vi "DimIndicators.dic_info_service.vi"(0 "controlRef":refnum<vi>, 2 "serviceName":string, 5 "error in (no error)":errorcluster) -> (14 "controlRef out":refnum<vi>, 19 "error out":errorcluster)   [LabVIEW 2015, in "DimIndicators.lvlib"]
doc: "Registers a control of one of the types in \"typedefs\" to a DIM service. If no longer used, a registered event should be unregistered using \"release service\"."
uses:
  DimIndicators.lvlib
  DimIndicators.numericType.ctl
  DimIndicators.numericArrayType.ctl
  DimIndicators.anyType.ctl
  DimIndicators.dataType.ctl
  DimIndicators.actionType.ctl
panel:
  in  "anyType":T1
  in  "numericArrayType":T2
  in  "numericType":T3
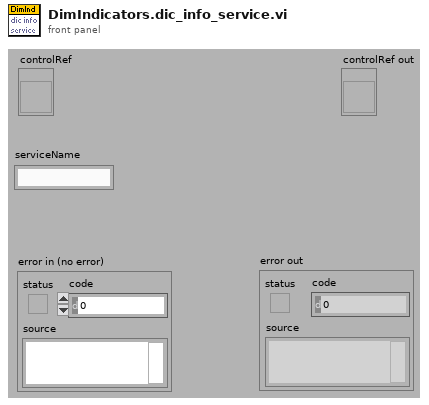
[diagram p1: front panel]
types:
  T1 = typedef "DimIndicators.lvlib/DimIndicators.anyType.ctl" = cluster{"data":string, "no link":bool, "quality":i32, "timeStamp":dbl}
  T2 = typedef "DimIndicators.lvlib/DimIndicators.numericArrayType.ctl" = cluster{"data":dbl[], "no link":bool, "quality":i32, "timeStamp":dbl}
  T3 = typedef "DimIndicators.lvlib/DimIndicators.numericType.ctl" = cluster{"data":dbl, "no link":bool, "quality":i32, "timeStamp":dbl}
  T4 = typedef "DimIndicators.lvlib/DimIndicators.dataType.ctl" = enum16{"unknown", "numeric", "numericArray", "any"}
  T5 = typedef "DimIndicators.lvlib/DimIndicators.actionType.ctl" = enum16{"dic_info_service", "dic_release_service", "init", "getControlRef", "getCallbackID", "close"}
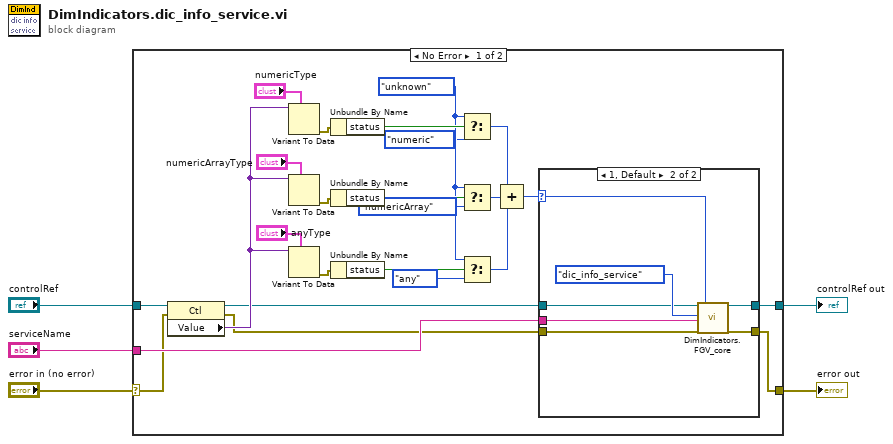
[diagram p0: block diagram]
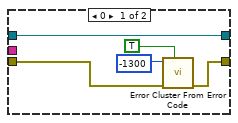
[diagram p2: hidden frame]
diagram:
  n1 = case shown="No Error" "error in (no error)" {
    selector: "error in (no error)" -> [w8 w44]
    tunnel: [w30 w44] -> w4
    tunnel: "serviceName" -> [w29 _]
    tunnel: "controlRef" -> [w28 w43]
    tunnel: [w9 w43] -> w1
    frame No Error {
      w17 = DimIndicators.dataType."unknown" ("actions")
      n2 = property on="Property Node" class="Ctl"(reference=w28, error in=w8) -> (reference out=w6:refnum<vi>, error out=w7:errorcluster, "Value"=w24:variant)
      n3 = Variant To Data(type="numericType", Variant=w24) -> (error out=w23:errorcluster)  [unwired: 1 in, 1 out]
      n4 = Variant To Data(type="numericArrayType", Variant=w24) -> (error out=w22:errorcluster)  [unwired: 1 in, 1 out]
      n5 = Variant To Data(type="anyType", Variant=w24) -> (error out=w21:errorcluster)  [unwired: 1 in, 1 out]
      n6 = Unbundle By Name(w23) -> ("status"=w20:bool)
      n7 = Unbundle By Name(w22) -> ("status"=w19:bool)
      n8 = Unbundle By Name(w21) -> ("status"=w18:bool)
      n9 = Select(t=w17, s=w20, f=DimIndicators.dataType."numeric") -> (s? t:f=w12:T4)
      n10 = Select(t=w17, s=w19, f=DimIndicators.dataType."numericArray") -> (s? t:f=w13:T4)
      n11 = Select(t=w17, s=w18, f=DimIndicators.dataType."any") -> (s? t:f=w11:T4)
      n12 = Compound Arithmetic op=unknown(w12, w13, w11) -> (w10:u16)
      n13 = case shown="1, Default" w10 {
        selector: w10 -> [_ w37]
        tunnel: w7 -> [w34 w42]
        tunnel: [w33 w41] -> w30
        tunnel: w29 -> [_ w40]
        tunnel: w6 -> [w35 w38]
        tunnel: [w35 w36] -> w9
        frame 0 {
          n14 = call <vilib>:"Error Cluster From Error Code.vi"("show call chain? (False)"=TRUE, "error in (no error)"=w34, "error code (0)"=-1300 ("code")) -> ("error out"=w33:errorcluster)  [unwired: 6 in]
        }
        frame 1, Default {
          n15 = call "DimIndicators.FGV_core.vi"("controlRef"=w38, "actions"=DimIndicators.actionType."dic_info_service", "serviceName"=w40, "error in (no error)"=w42, "dataType"=w37) -> ("controlRef out"=w36:refnum<vi>, "error out"=w41:errorcluster)  [unwired: 11 in, 2 out]
        }
      }
    }
    frame Error {
    }
  }
  "error out" <- w4
  "controlRef out" <- w1
